vi "Error Handler.vi"(8 "error in (no error)":errorcluster) -> (0 "error out":errorcluster)   [LabVIEW 2016, in "Shared Variable Interface.lvlib"]
uses:
  Shared Variable Interface.lvlib
  <vilib>/ErrorRing/Error Ring.xnode
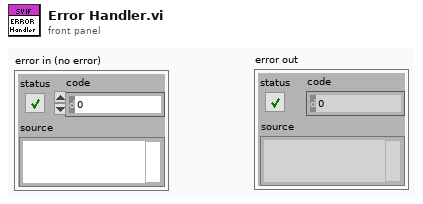
[diagram p1: front panel]
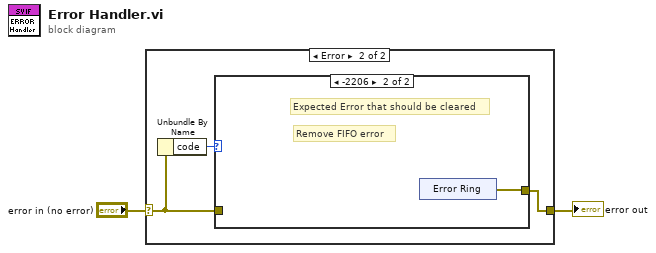
[diagram p0: block diagram]
diagram:
  n1 = case shown="Error" "error in (no error)" {
    selector: "error in (no error)" -> [w3 w5]
    tunnel: [w3 w4] -> w1
    frame No Error {
    }
    frame Error {
      n2 = Unbundle By Name(w5) -> ("code"=w6:i32)
      n3 = case shown="-2206" w6 {
        tunnel: w5 -> [w7 _]
        tunnel: [w7 w8] -> w4
        frame 0, Default {
        }
        frame -2206 {
          # "Remove FIFO error"
          # "Expected Error that should be cleared"
          n4 = xnode "Error Ring"() -> ("error out"=w8:errorcluster)
        }
      }
    }
  }
  "error out" <- w1
